vi "Engine Daemon Async.vi"(8 "error in (no error)":errorcluster, 10 "Daemon Notifier":refnum<notifier>, 11 "TSEngine in":refnum<class "Engine.lvclass">) -> ()   [LabVIEW 2020, in "TSS.lvlib" / "Engine.lvclass"]
uses:
  Engine.lvclass
  Engine.lvclass/Engine.ctl
  VariableContainer/VariableContainer.lvclass
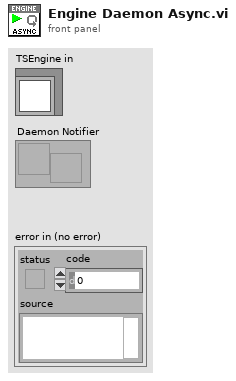
[diagram p1: front panel]
types:
  T1 = typedef "TSS.lvlib/Engine.lvclass/Events.ctl" = cluster{"Stop Deamon":refnum<user-event>, "Create Variable Container":refnum<user-event>}
  T2 = typedef "TSS.lvlib/Engine.lvclass/Variable Container Type.ctl" = enum16{"StationGlobals", "TemporaryGlobals", "NewPropertyObject"}
  T3 = typedef "TSS.lvlib/VariableContainer.lvclass/Session Handle.ctl" = refnum<data-value>
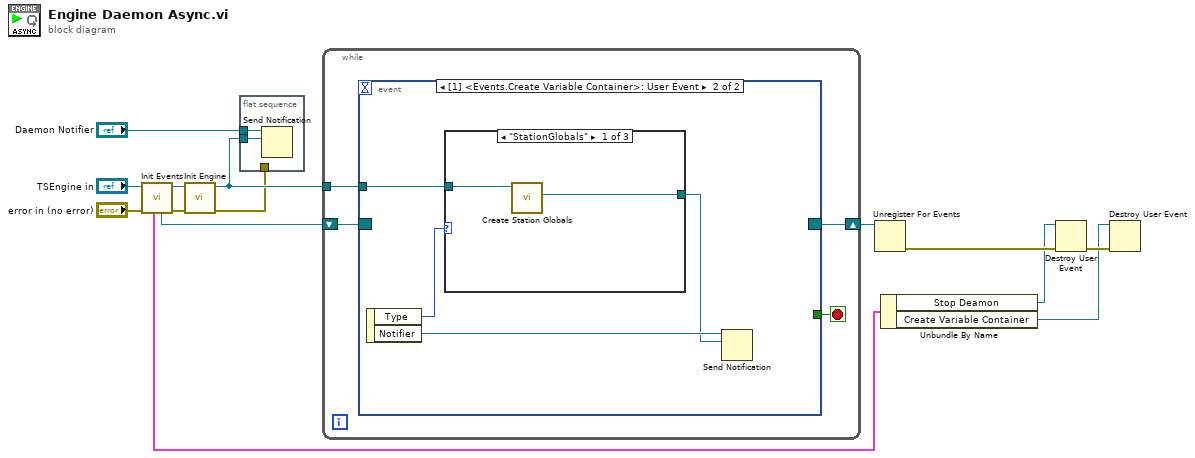
[diagram p0: block diagram]
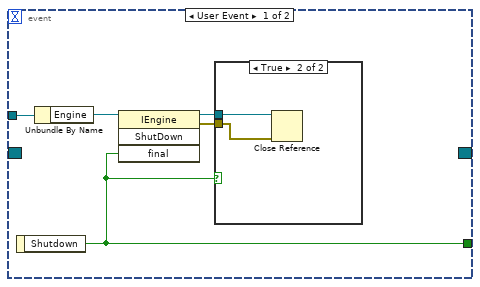
[diagram p2: hidden frame]
diagram:
  n1 = call "Init Events.vi"("error in (no error)"="error in (no error)", "TSEngine in"="TSEngine in") -> ("error out"=w8:errorcluster, "TSEngine out"=w9:refnum<class "Engine.lvclass">, "Event Reg"=w6:refnum<event-registration>, "Events"=w4:T1)  [unwired: 6 in]
  n2 = call "Init Engine.vi"("error in (no error)"=w8, "TSEngine in"=w9) -> ("error out"=w7:errorcluster, "TSEngine out"=w12:refnum<class "Engine.lvclass">)  [unwired: 8 in]
  n3 = flat-sequence {
    tunnel: "Daemon Notifier" -> [w16]
    tunnel: w12 -> [w15]
    tunnel: w7 -> [_]
    frame #0 {
      n4 = Send Notification(notification=w15, notifier=w16) -> ()  [unwired: 1 in, 2 out]
    }
  }
  n5 = while {
    shift-right: [w19] -> w13
    shift-left: w6 -> [w20]
    tunnel: w12 -> [w17]
    stop <- w18 stop-if-true
    n6 = event shown="[1] <Events.Create Variable Container>: User Event" {
      selector: w20 -> [_ _]
      dyn-events: [_ _] -> w19
      timeout: _ -> [_ _]
      tunnel: [w23 _] -> w18
      tunnel: w17 -> [w25 w30]
      event User Event {
        n7 = event-data() -> ("Shutdown"=w23:bool)  [unwired: 1 in]
        n8 = Unbundle By Name(w25) -> ("Engine"=w24:refnum<k7>)
        n9 = invoke class="IEngine" method="ShutDown"(reference=w24, "final"=w23) -> (reference out=w22:refnum<k7>, error out=w21:errorcluster)  [unwired: 2 in, 2 out]
        n10 = case shown="True" w23 {
          tunnel: w22 -> [_ w27]
          tunnel: w21 -> [_ w26]
          frame False {
          }
          frame True {
            n11 = Close Reference(reference=w27, error in (no error)=w26) -> ()  [unwired: 1 out]
          }
        }
      }
      event User Event {
        n12 = event-data() -> ("Type"=w31:T2, "Notifier"=w29:refnum<notifier>)  [unwired: 1 in]
        n13 = case shown="\"StationGlobals\"" w31 {
          tunnel: w30 -> [w33 _ _]
          tunnel: [w32 _ _] -> w28
          frame "StationGlobals" {
            n14 = call "Create Station Globals.vi"("TSEngine in"=w33) -> ("StationGlobals"=w32:T3)  [unwired: 8 in, 2 out]
          }
          frame "TemporaryGlobals" {
          }
          frame "NewPropertyObject" {
          }
        }
        n15 = Send Notification(notification=w28, notifier=w29) -> ()  [unwired: 1 in, 2 out]
      }
    }
  }
  n16 = Unregister For Events(event registration refnum=w13) -> (error out=w5:errorcluster)  [unwired: 1 in]
  n17 = Unbundle By Name(w4) -> ("Stop Deamon"=w3:refnum<user-event>, "Create Variable Container"=w1:refnum<user-event>)
  n18 = Destroy User Event(user event=w3, error in=w5) -> (error out=w2:errorcluster)
  n19 = Destroy User Event(user event=w1, error in=w2) -> ()  [unwired: 1 out]
